vi "Time in ms to Counter Value.vi"(11 "time (ms)":dbl) -> (3 "counter value":dbl)   [LabVIEW 2017, in "Engine Simulation Toolkit System Explorer.lvlib"]
uses:
  Engine Simulation Toolkit System Explorer.lvlib
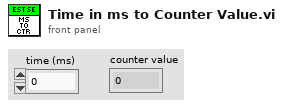
[diagram p1: front panel]
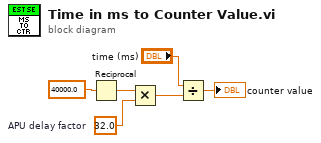
[diagram p0: block diagram]
diagram:
  w4 = 32.0  # APU delay factor
  n1 = Reciprocal(x=40000.0) -> (1/x=w5:dbl)
  n2 = Multiply(x=w5, y=w4) -> (x*y=w2:dbl)
  n3 = Divide(x="time (ms)", y=w2) -> (x/y=→"counter value":dbl)
